vi "Main.vi"() -> ()   [LabVIEW 2022 SP3]
doc: "This template is for the Queued Message Handler design pattern.\n\nThe Event Handling Loop generates messages based on user interface actions.\n\nThe Message Handling Loop processes messages generated by the Event Handling Loop, or by other messages. The messages are string values, so new messages can be added easily to the Message Cases case structure in the Message Handling Loop. Each message cluster can also provide an optional value for Message Data, which is a variant that can be converted to whatever message-specific data is required."
uses:
  controls/UI Data.ctl
  controls/UI State.ctl
  controls/Config.ctl
  support/Message Queue/Enqueue Message (Single).vi
  support/Message Queue/Enqueue Message (Array).vi
  <vilib>/Utility/error.llb/Error Cluster From Error Code.vi
  <vilib>/ErrorRing/Error Ring.xnode
  support/Message Queue/Message Queue.lvlib
  support/User Event - Stop/User Event - Stop.lvlib
  Logging/Logging.lvlib
panel:
  out "PWM Value":dbl
  out "Temperature":dbl
  out "Stop":bool=TRUE
  out "Run":bool=TRUE
  out "PWM":dbl(knob) scale=0.0..255.0
  out "Hibák":errorcluster
  out "Waveform Chart":waveform(dbl)[](graph)
  out "Output":cluster{cluster{"Xi":dbl, "Yi":dbl}[]}[](graph)
  out "Error":cluster{cluster{"Xi":dbl, "Yi":dbl}[]}[](graph)
  out "Temperature":cluster{cluster{"Xi":dbl, "Yi":dbl}[]}[](graph)
  in  "Settings":bool
  out "Display":string
  in  "Stop":bool
  in  "Start":bool
  in  "Exit":bool
  # "°C"
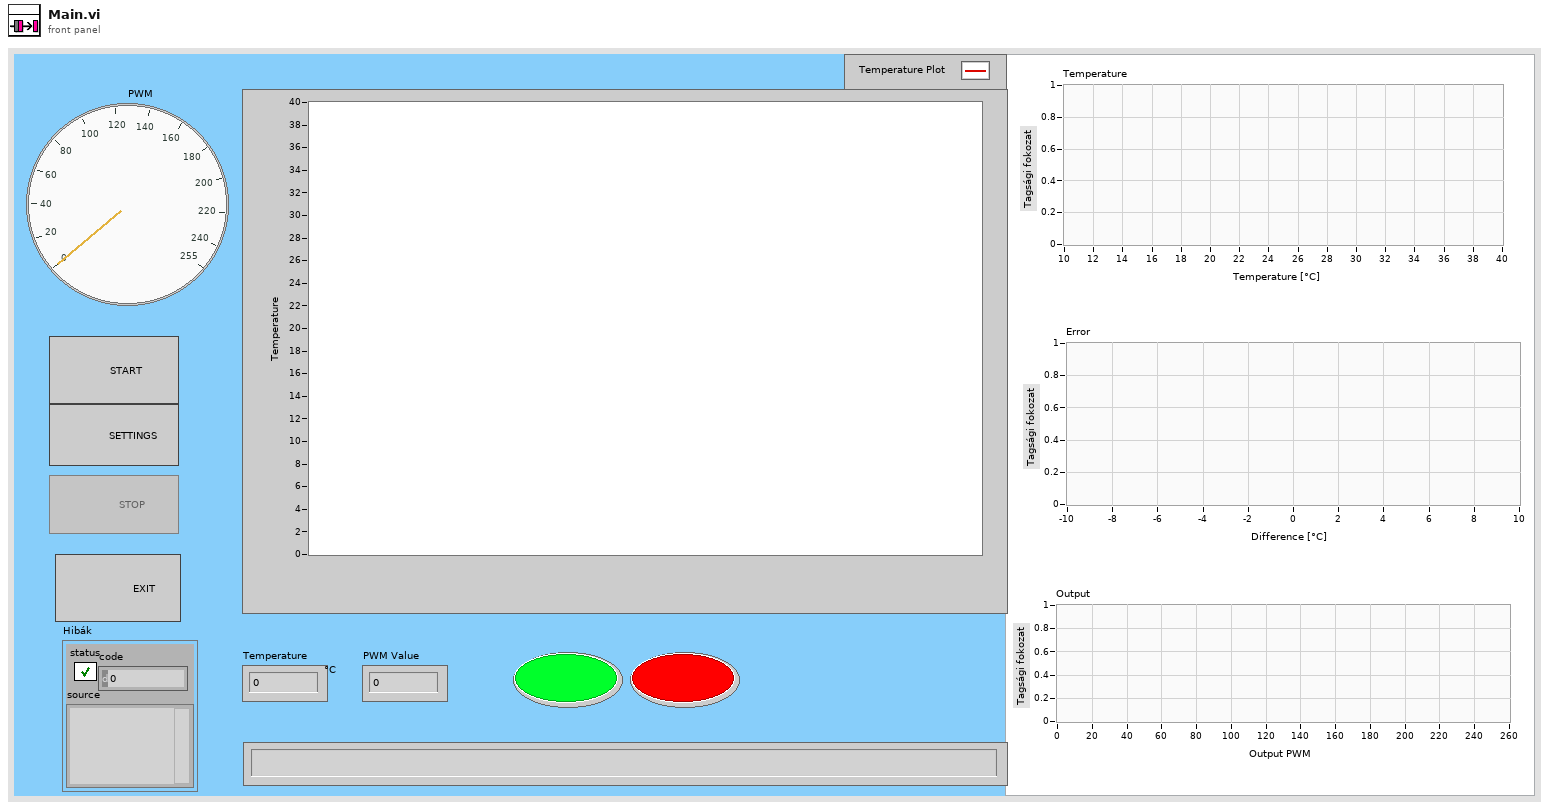
[diagram p1: front panel]
types:
  T1 = typedef "Config.ctl" = cluster{"Hardware":cluster{"VISA resource name":refnum<visa-resource-name>}, "Logging":cluster{"tdms file out":refnum<k34>, "base path":path}, "Set Temp":cluster{"Numeric":dbl}}
  T2 = typedef "UI State.ctl" = enum16{"Idle", "Acquiring and logging", "Waiting for Exit", "Waiting for Stop"}
  T3 = typedef "UI Data.ctl" = cluster{"Boolean <Replace Me>":bool, "String":string, "Numeric <Replace Me>":dbl, "Start ref":refnum<vi>, "Stop ref":refnum<vi>, "Data Display Ref":refnum<vi>, "Exit Button Ref":refnum<vi>, "Settings ref":refnum<vi>}
  T4 = typedef "Message Queue.lvlib/All Message Queues.ctl" = cluster{"UI":refnum<queue>, "Acquisition":refnum<queue>, "Logging":refnum<queue>}
  T5 = cluster{"Hardware":cluster{"VISA resource name":refnum<visa-resource-name>}, "Logging":cluster{"tdms file out":refnum<k34>, "base path":path}, "Set Temp":cluster{"Numeric":dbl}}
  T6 = cluster{"tdms file out":refnum<k34>, "base path":path}
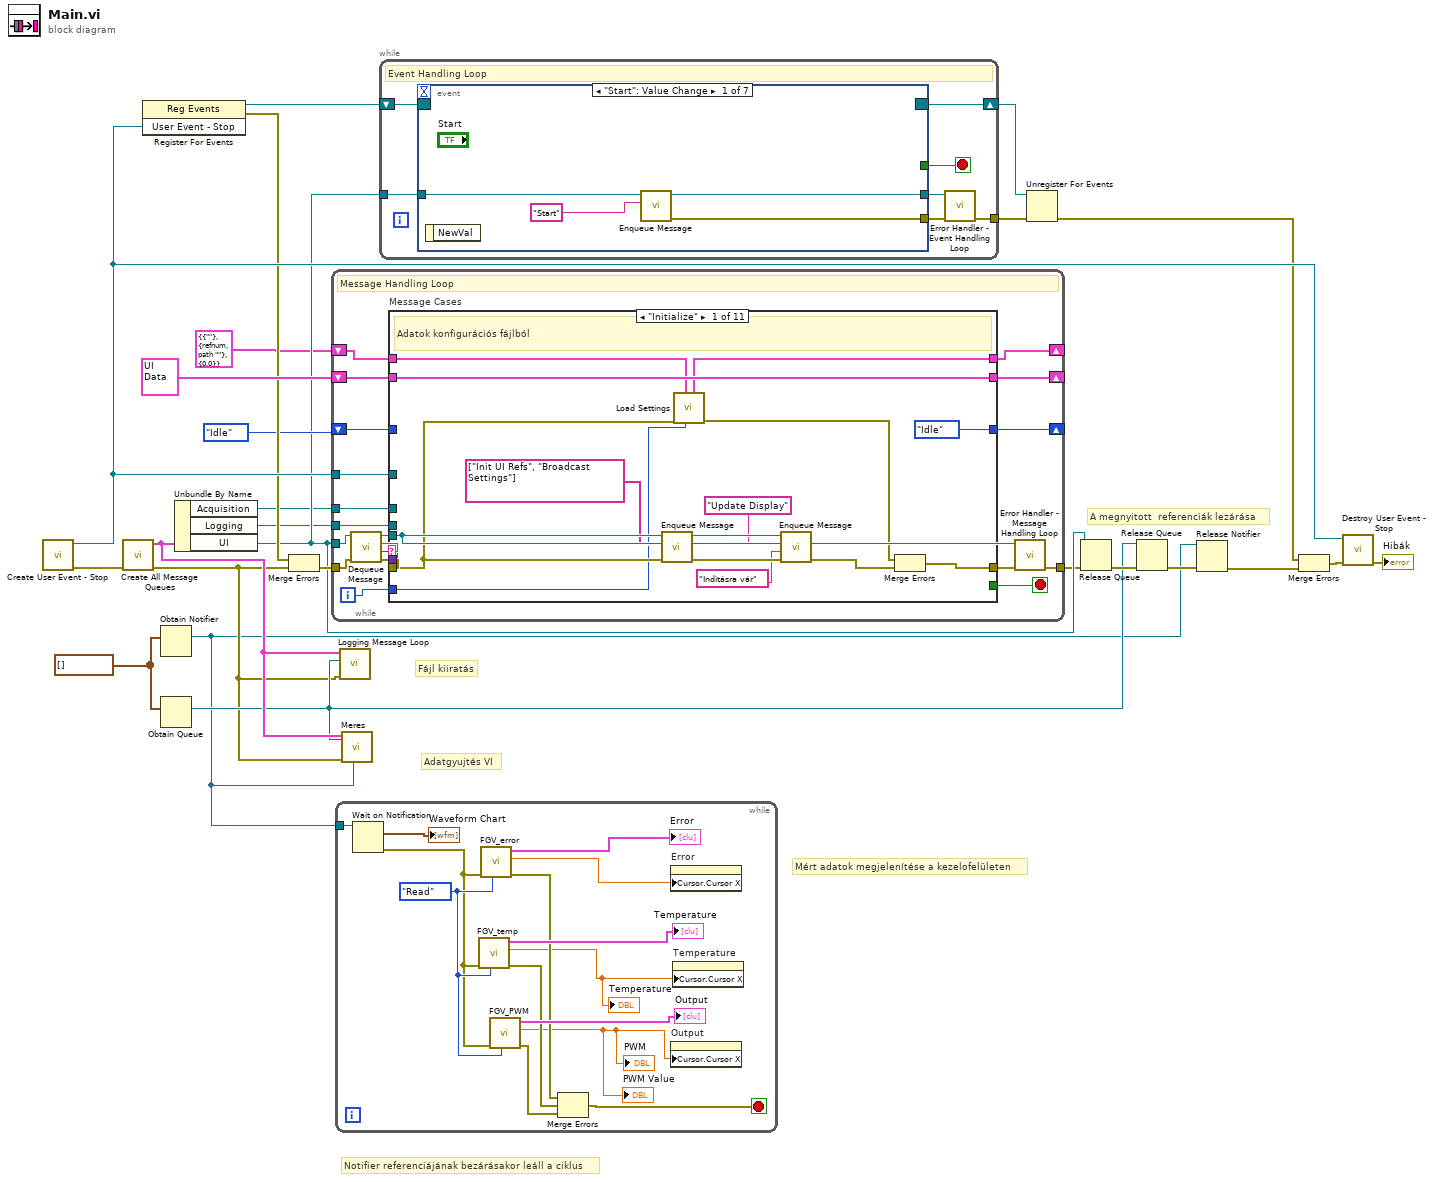
[diagram p0: block diagram]
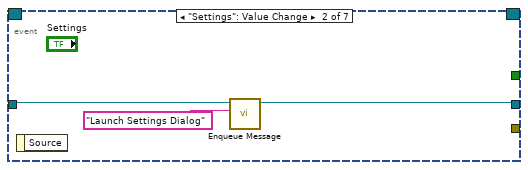
[diagram p2: hidden frame]
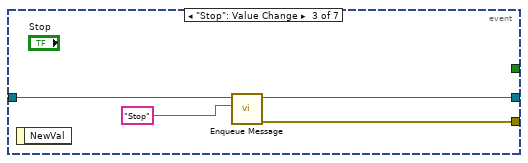
[diagram p3: hidden frame]
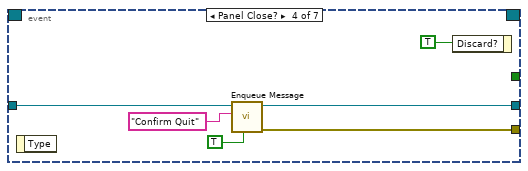
[diagram p4: hidden frame]
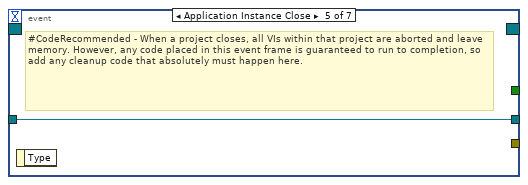
[diagram p5: hidden frame]
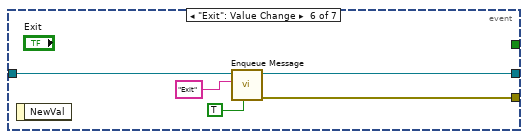
[diagram p6: hidden frame]
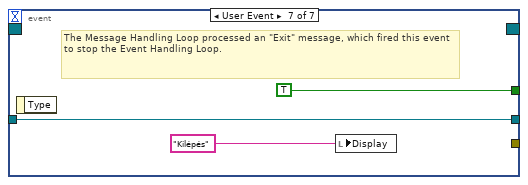
[diagram p7: hidden frame]
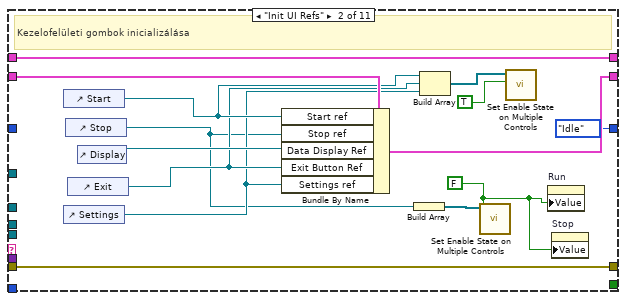
[diagram p8: hidden frame]
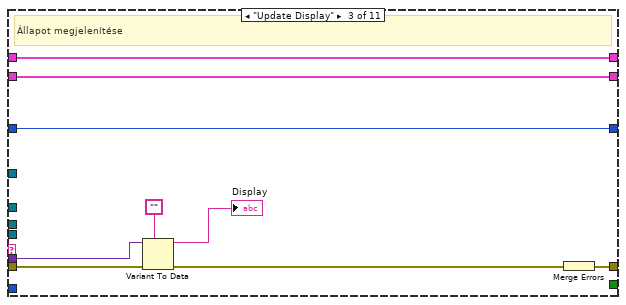
[diagram p9: hidden frame]
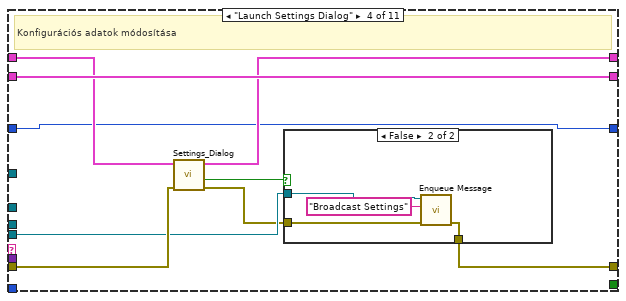
[diagram p10: hidden frame]
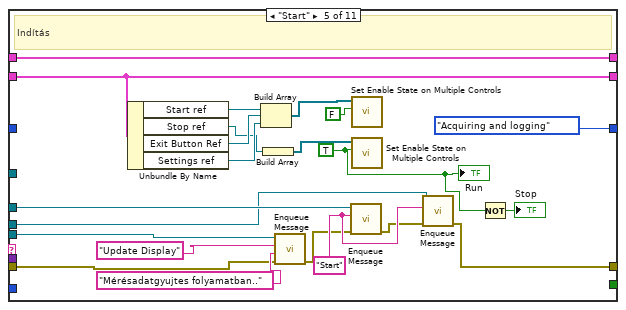
[diagram p12: hidden frame]
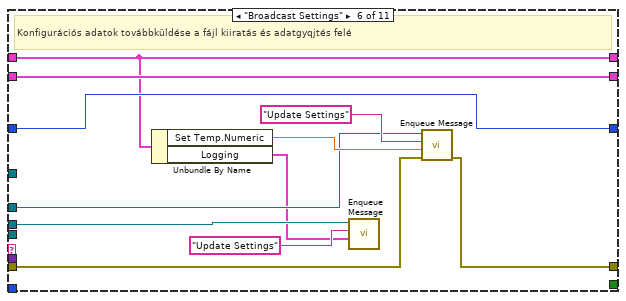
[diagram p13: hidden frame]
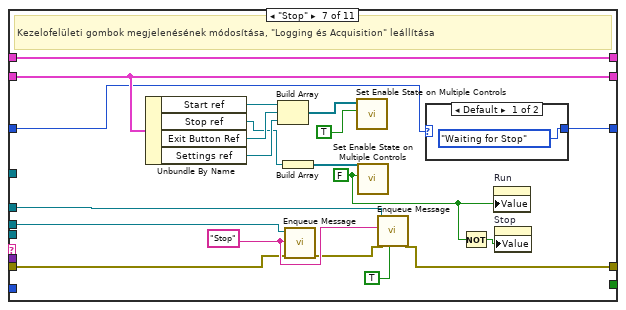
[diagram p14: hidden frame]
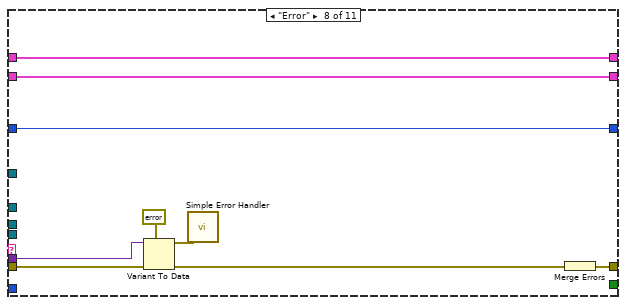
[diagram p16: hidden frame]
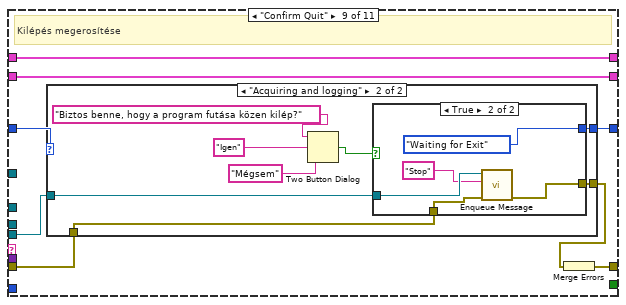
[diagram p17: hidden frame]
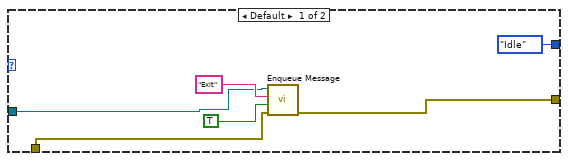
[diagram p18: hidden frame]
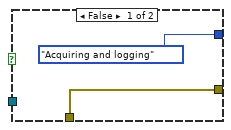
[diagram p19: hidden frame]
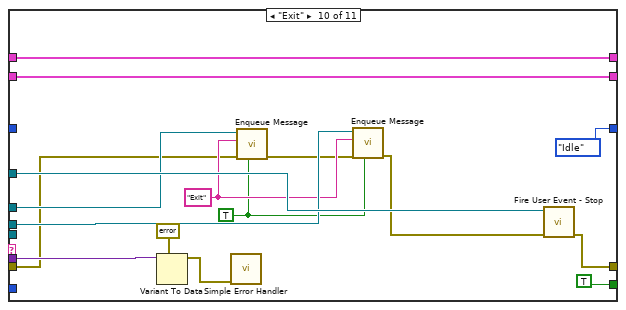
[diagram p20: hidden frame]
diagram:
  w9 = waveform(dbl)[] []
  # "Notifier referenciájának bezárásakor leáll a ciklus"
  # "Fájl kiiratás"
  # "Adatgyujtés VI"
  # "Mért adatok megjelenítése a kezelofelületen"
  # "A megnyitott  referenciák lezárása"
  n1 = call "Create User Event - Stop.vi"() -> ("error out"=w25:errorcluster, "User Event - Stop"=w19:refnum<user-event>)  [unwired: 10 in]
  n2 = call "Create All Message Queues.vi"("error in (no error)"=w25) -> ("error out"=w4:errorcluster, "Message Queues out"=w6:T4)  [unwired: 9 in]
  n3 = register-events(w19) -> (reference out=w20:refnum<event-registration>, error out=w17:errorcluster)  [unwired: 2 in]
  n4 = Obtain Notifier(notification data type=w9) -> (notifier out=w3:refnum<notifier>)  [unwired: 3 in, 2 out]
  n5 = Obtain Queue(element data type=w9) -> (queue out=w5:refnum<queue>)  [unwired: 4 in, 2 out]
  n6 = Unbundle By Name(w6) -> ("Acquisition"=w12:refnum<queue>, "Logging"=w11:refnum<queue>, "UI"=w15:refnum<queue>)
  n7 = Merge Errors(w17, w4) -> (w18:errorcluster)
  n8 = while {
    tunnel: w15 -> [w36]
    shift-right: [w43] -> _
    shift-left: T3 {"Boolean <Replace Me>"=FALSE, "String"="", "Numeric <Replace Me>"=0.0, "Start ref"=refnum, "Stop ref"=refnum, "Data Display Ref"=refnum, "Exit Button Ref"=refnum, "Settings ref"=refnum} ("Data Cluster") -> [w44]
    tunnel: w19 -> [w41]
    tunnel: w18 -> [w40]
    tunnel: [w34] -> w10
    shift-right: [w32] -> _
    shift-left: UI_State."Idle" -> [w31]
    shift-right: [w30] -> _
    shift-left: T1 {"Hardware"={"VISA resource name"=""}, "Logging"={"tdms file out"=refnum, "base path"=path ""}, "Set Temp"={"Numeric"=0.0}} -> [w29]
    tunnel: w12 -> [w28]
    tunnel: w11 -> [w27]
    i -> [w26]
    stop <- w42 stop-if-true
    # "Message Handling Loop"
    n9 = call "Dequeue Message.vi"("error in (no error)"=w40, "Message Queue"=w36) -> ("error out"=w39:errorcluster, "Message Data"=w37:variant, "Message"=w38:string, "dup Message Queue"=w35:refnum<queue>)  [unwired: 6 in]
    n10 = case "Message Cases" shown="\"Initialize\"" w38 {
      selector: w38 -> [_ _ _ _ _ _ _ _ _ _ w208]
      tunnel: w35 -> [w56 _ _ w86 w109 _ _ _ w164 _ _]
      tunnel: w39 -> [w48 w63 w80 w88 w106 w124 w136 w160 w162 w193 _]
      tunnel: [w47 w63 w81 w84 w99 w123 w134 w154 w167 w198 w209] -> w33
      tunnel: w44 -> [w59 w73 w82 w91 w118 w129 w149 w159 w168 w205 w210]
      tunnel: [w59 w64 w82 w91 w118 w129 w149 w159 w168 w205 w210] -> w43
      tunnel: [_ _ _ _ _ _ _ _ _ TRUE _] -> w42
      tunnel: w37 -> [_ _ w79 _ _ _ _ w158 _ w200 _]
      tunnel: w41 -> [_ _ _ _ _ _ _ _ _ w203 _]
      tunnel: [UI_State."Idle" UI_State."Idle" w74 w83 UI_State."Acquiring and logging" w128 w140 w153 w163 UI_State."Idle" w206] -> w32
      tunnel: w31 -> [_ _ w74 w83 _ w128 w141 w153 w165 _ w206]
      tunnel: [w49 w62 w75 w89 w105 w122 w139 w152 w166 w197 w207] -> w30
      tunnel: w29 -> [w50 w62 w75 w90 w105 w122 w139 w152 w166 w197 w207]
      tunnel: w28 -> [_ _ _ _ w104 w125 w138 _ _ w196 _]
      tunnel: w27 -> [_ _ _ _ w103 w121 w132 _ _ w195 _]
      tunnel: w26 -> [w45 _ _ _ _ _ _ _ _ _ _]
      frame "Initialize" {
        # "Adatok konfigurációs fájlból"
        n11 = call-poly "Enqueue Message.vi"("error in (no error)"=w48, "Message Array"=string[] ["Init UI Refs", "Broadcast Settings"], "Message Queue"=w56) -> ("error out"=w58:errorcluster, "dup Message Queue"=w55:refnum<queue>)  [unwired: 7 in]
        n12 = call "Load Settings.vi"("Elso?"=w45, "Config"=w50, "error constant"=w48) -> ("error constant 2"=w46:errorcluster, "Config 2"=w49:T5)  [unwired: 7 in]
        n13 = call-poly "Enqueue Message.vi"("error in (no error)"=w58, "Message Data"="Inditásra vár" ("Message"), "Message"="Update Display", "Message Queue"=w55) -> ("error out"=w57:errorcluster)  [unwired: 6 in, 1 out]
        n14 = Merge Errors(w46, w57) -> (w47:errorcluster)
      }
      frame "Init UI Refs" {
        w60 = FALSE ("Enable?")
        # "Kezelofelületi gombok inicializálása"
        n15 = control-ref of="Start"() -> (w71:refnum<vi>)
        n16 = control-ref of="Settings"() -> (w69:refnum<vi>)
        n17 = control-ref of="Stop"() -> (w68:refnum<vi>)
        n18 = control-ref of="Exit"() -> (w70:refnum<vi>)
        n19 = control-ref of="Display"() -> (w72:refnum<vi>)
        n20 = Bundle By Name(cluster=w73, "Start ref"=w71, "Stop ref"=w68, "Data Display Ref"=w72, "Exit Button Ref"=w70, "Settings ref"=w69) -> (w64:T3)
        n21 = Build Array(w68) -> (w67:refnum<vi>[])
        n22 = Build Array(w71, w70, w69) -> (w66:refnum<vi>[])
        n23 = call "Set Enable State on Multiple Controls.vi"("Enable?"=w60, "Controls"=w67) -> ()  [unwired: 10 in]
        n24 = call "Set Enable State on Multiple Controls.vi"("Enable?"=TRUE, "Controls"=w66) -> ()  [unwired: 10 in]
        n25 = property on="Run" class="Bool (strict)"("Value"=w60) -> ()  [unwired: 2 in, 2 out]
        n26 = property on="Stop" class="Bool (strict)"("Value"=w60) -> ()  [unwired: 2 in, 2 out]
      }
      frame "Update Display" {
        # "Állapot megjelenítése"
        n27 = Variant To Data(error in=w80, type="", Variant=w79) -> (data=→"Display":string, error out=w77:errorcluster)
        n28 = Merge Errors(w77) -> (w81:errorcluster)
      }
      frame "Launch Settings Dialog" {
        # "Konfigurációs adatok módosítása"
        n29 = call "Settings_Dialog.vi"("error IO 2"=w88, "Settings in"=w90) -> ("error IO"=w85:errorcluster, "Cancelled"=w87:bool, "Settings out"=w89:T1)  [unwired: 7 in]
        n30 = case shown="False" w87 {
          tunnel: w86 -> [_ w95]
          tunnel: w85 -> [w92 w94]
          tunnel: [w92 w93] -> w84
          frame True {
          }
          frame False {
            n31 = call-poly "Enqueue Message.vi"("error in (no error)"=w94, "Message"="Broadcast Settings", "Message Queue"=w95) -> ("error out"=w93:errorcluster)  [unwired: 7 in, 1 out]
          }
        }
      }
      frame "Start" {
        w102 = "Start" ("Message")
        w98 = TRUE ("Enable?")
        # "Indítás"
        n32 = Unbundle By Name(w118) -> ("Start ref"=w116:refnum<vi>, "Stop ref"=w111:refnum<vi>, "Exit Button Ref"=w115:refnum<vi>, "Settings ref"=w114:refnum<vi>)
        n33 = Build Array(w116, w115, w114) -> (w113:refnum<vi>[])
        n34 = Build Array(w111) -> (w112:refnum<vi>[])
        n35 = call-poly "Enqueue Message.vi"("error in (no error)"=w106, "Message Data"="Mérésadatgyujtes folyamatban.." ("Message"), "Message"="Update Display", "Message Queue"=w109) -> ("error out"=w101:errorcluster)  [unwired: 6 in, 1 out]
        n36 = call-poly "Enqueue Message.vi"("error in (no error)"=w101, "Message"=w102, "Message Queue"=w104) -> ("error out"=w100:errorcluster)  [unwired: 7 in, 1 out]
        n37 = call "Set Enable State on Multiple Controls.vi"("Enable?"=FALSE, "Controls"=w113) -> ()  [unwired: 10 in]
        n38 = call "Set Enable State on Multiple Controls.vi"("Enable?"=w98, "Controls"=w112) -> ()  [unwired: 10 in]
        n39 = call-poly "Enqueue Message.vi"("error in (no error)"=w100, "Message"=w102, "Message Queue"=w103) -> ("error out"=w99:errorcluster)  [unwired: 7 in, 1 out]
        n40 = Not(x=w98) -> (.not. x?=→"Stop":bool)
        "Run" <- w98
      }
      frame "Broadcast Settings" {
        # "Konfigurációs adatok továbbküldése a fájl kiiratás és adatgyqjtés felé"
        n41 = Unbundle By Name(w122) -> ("Set Temp.Numeric"=w127:dbl, "Logging"=w119:T6)
        n42 = call-poly "Enqueue Message.vi"("Message Data"=w119, "Message"="Update Settings", "Message Queue"=w121) -> ()  [unwired: 7 in, 2 out]
        n43 = call-poly "Enqueue Message.vi"("error in (no error)"=w124, "Message Data"=w127, "Message"="Update Settings", "Message Queue"=w125) -> ("error out"=w123:errorcluster)  [unwired: 6 in, 1 out]
      }
      frame "Stop" {
        w137 = "Stop" ("Message")
        w130 = FALSE ("Enable?")
        # "Kezelofelületi gombok megjelenésének módosítása, \"Logging és Acquisition\" leállítása"
        n44 = Unbundle By Name(w149) -> ("Start ref"=w148:refnum<vi>, "Stop ref"=w144:refnum<vi>, "Exit Button Ref"=w147:refnum<vi>, "Settings ref"=w146:refnum<vi>)
        n45 = Build Array(w148, w147, w146) -> (w145:refnum<vi>[])
        n46 = Build Array(w144) -> (w143:refnum<vi>[])
        n47 = call-poly "Enqueue Message.vi"("error in (no error)"=w136, "Message"=w137, "Message Queue"=w132) -> ("error out"=w135:errorcluster)  [unwired: 7 in, 1 out]
        n48 = call "Set Enable State on Multiple Controls.vi"("Enable?"=TRUE, "Controls"=w145) -> ()  [unwired: 10 in]
        n49 = call "Set Enable State on Multiple Controls.vi"("Enable?"=w130, "Controls"=w143) -> ()  [unwired: 10 in]
        n50 = call-poly "Enqueue Message.vi"("Priority Message? (F)"=TRUE, "error in (no error)"=w135, "Message"=w137, "Message Queue"=w138) -> ("error out"=w134:errorcluster)  [unwired: 6 in, 1 out]
        n51 = case shown="Default" w141 {
          selector: w141 -> [_ w151]
          tunnel: [UI_State."Waiting for Stop" w151] -> w140
          frame Default {
          }
          frame "Waiting for Exit" {
          }
        }
        n52 = Not(x=w130) -> (.not. x?=w131:bool)
        n53 = property on="Run" class="Bool (strict)"("Value"=w130) -> ()  [unwired: 2 in, 2 out]
        n54 = property on="Stop" class="Bool (strict)"("Value"=w131) -> ()  [unwired: 2 in, 2 out]
      }
      frame "Error" {
        n55 = Variant To Data(error in=w160, type=errorcluster {"status"=FALSE, "code"=0, "source"=""} ("error constant"), Variant=w158) -> (data=w156:errorcluster, error out=w155:errorcluster)
        n56 = call <vilib>:"Simple Error Handler.vi"("error in (no error)"=w156) -> ()  [unwired: 4 in, 5 out]
        n57 = Merge Errors(w155) -> (w154:errorcluster)
      }
      frame "Confirm Quit" {
        # "Kilépés megerosítése"
        n58 = case shown="\"Acquiring and logging\"" w165 {
          tunnel: w164 -> [w172 w178]
          tunnel: [UI_State."Idle" w177] -> w163
          tunnel: w162 -> [w170 w176]
          tunnel: [w169 w175] -> w161
          frame Default {
            n59 = call-poly "Enqueue Message.vi"("error in (no error)"=w170, "Message Data"=TRUE ("Priority Message? (F)"), "Message"="Exit", "Message Queue"=w172) -> ("error out"=w169:errorcluster)  [unwired: 6 in, 1 out]
          }
          frame "Acquiring and logging" {
            n60 = Two Button Dialog(message="Biztos benne, hogy a program futása közen kilép?", 1:"Mégsem" ("F button name (\"Cancel\")"), 2:"Igen" ("T button name (\"OK\")")) -> (T button?=w179:bool)
            n61 = case shown="True" w179 {
              tunnel: w178 -> [_ w189]
              tunnel: [UI_State."Acquiring and logging" UI_State."Waiting for Exit"] -> w177
              tunnel: [w183 w185] -> w175
              tunnel: w176 -> [w183 w186]
              frame False {
              }
              frame True {
                n62 = call-poly "Enqueue Message.vi"("error in (no error)"=w186, "Message"="Stop", "Message Queue"=w189) -> ("error out"=w185:errorcluster)  [unwired: 7 in, 1 out]
              }
            }
          }
        }
        n63 = Merge Errors(w161) -> (w167:errorcluster)
      }
      frame "Exit" {
        w190 = TRUE ("Priority Message? (F)")
        w194 = "Exit" ("Message")
        n64 = Variant To Data(type=errorcluster {"status"=FALSE, "code"=0, "source"=""} ("error constant"), Variant=w200) -> (data=w201:errorcluster)  [unwired: 1 in, 1 out]
        n65 = call <vilib>:"Simple Error Handler.vi"("error in (no error)"=w201) -> ()  [unwired: 4 in, 5 out]
        n66 = call-poly "Enqueue Message.vi"("Priority Message? (F)"=w190, "error in (no error)"=w193, "Message"=w194, "Message Queue"=w196) -> ("error out"=w192:errorcluster)  [unwired: 6 in, 1 out]
        n67 = call-poly "Enqueue Message.vi"("Priority Message? (F)"=w190, "error in (no error)"=w192, "Message"=w194, "Message Queue"=w195) -> ("error out"=w191:errorcluster)  [unwired: 6 in, 1 out]
        n68 = call "Fire User Event - Stop.vi"("error in (no error)"=w191, "User Event - Stop"=w203) -> ("error out"=w198:errorcluster)  [unwired: 9 in]
      }
      frame Default {
        n69 = xnode "Error Ring"("parameter 0"=w208) -> ("error out"=w209:errorcluster)
      }
    }
    n70 = call "Error Handler - Message Handling Loop.vi"("error in (no error)"=w33, "Message Queue"=w35) -> ("dup error in"=w34:errorcluster)  [unwired: 8 in, 1 out]
  }
  n71 = while {
    tunnel: w3 -> [w231]
    stop <- w220 stop-if-true
    w225 = enum16{"Read", "Write"}."Read" ("R/W")
    n72 = Wait on Notification(notifier=w231) -> (notification=→"Waveform Chart":waveform(dbl)[], error out=w224:errorcluster)  [unwired: 3 in, 2 out]
    n73 = call "FGV_temp.vi"("R/W"=w225, "error"=w224) -> ("error  out"=w222:errorcluster, "Value out"=w219:dbl, "Temp out"=→"Temperature":cluster{cluster{"Xi":dbl, "Yi":dbl}[]}[])  [unwired: 7 in]
    "Temperature" <- w219
    n74 = call "FGV_error.vi"("R/W"=w225, "error"=w224) -> ("error  out"=w223:errorcluster, "Value out"=w228:dbl, "FuzzyError out"=→"Error":cluster{cluster{"Xi":dbl, "Yi":dbl}[]}[])  [unwired: 7 in]
    n75 = call "FGV_PWM.vi"("R/W"=w225, "error"=w224) -> ("error  out"=w221:errorcluster, "Value out"=w218:dbl, "PWM out"=→"Output":cluster{cluster{"Xi":dbl, "Yi":dbl}[]}[])  [unwired: 7 in]
    "PWM" <- w218
    "PWM Value" <- w218
    n76 = Merge Errors(w223, w222, w221) -> (w220:errorcluster)
    n77 = property on="Error" class="XYGraph (strict)"("Cursor.Cursor X"=w228) -> ()  [unwired: 2 in, 2 out]
    n78 = property on="Output" class="XYGraph (strict)"("Cursor.Cursor X"=w218) -> ()  [unwired: 2 in, 2 out]
    n79 = property on="Temperature" class="XYGraph (strict)"("Cursor.Cursor X"=w219) -> ()  [unwired: 2 in, 2 out]
  }
  n80 = call "Logging Message Loop.vi"("error in (no error)"=w4, "Data Queue"=w5, "Message Queues"=w6) -> ()  [unwired: 8 in, 1 out]
  n81 = call "Meres.vi"("notifier"=w3, "queue"=w5, "error in"=w4, "Message Queues"=w6) -> ()  [unwired: 7 in, 1 out]
  n82 = while {
    tunnel: w15 -> [w238]
    shift-right: [w236] -> w23
    shift-left: w20 -> [w237]
    tunnel: [w232] -> w21
    stop <- w234 stop-if-true
    # "Event Handling Loop"
    n83 = event shown="[0] \"Start\": Value Change" {
      selector: w237 -> [_ _ _ _ _ _ _]
      dyn-events: [_ _ _ _ _ _ _] -> w236
      timeout: _ -> [_ _ _ _ _ _ _]
      tunnel: [_ _ _ _ _ _ TRUE ("Discard?")] -> w234
      tunnel: w238 -> [w242 w245 w249 w254 w256 w261 w264]
      tunnel: [w239 _ w246 w253 _ w260 _] -> w235
      tunnel: [w241 w243 w248 w252 w256 w259 w264] -> w233
      event "Start": Value Change {
        n84 = event-data() -> ()  [unwired: 1 in, 1 out]
        n85 = call-poly "Enqueue Message.vi"("Message"="Start", "Message Queue"=w242) -> ("error out"=w239:errorcluster, "dup Message Queue"=w241:refnum<queue>)  [unwired: 8 in]
      }
      event "Settings": Value Change {
        n86 = event-data() -> ()  [unwired: 1 in, 1 out]
        n87 = call-poly "Enqueue Message.vi"("Message"="Launch Settings Dialog", "Message Queue"=w245) -> ("dup Message Queue"=w243:refnum<queue>)  [unwired: 8 in, 1 out]
      }
      event "Stop": Value Change {
        n88 = event-data() -> ()  [unwired: 1 in, 1 out]
        n89 = call-poly "Enqueue Message.vi"("Message"="Stop", "Message Queue"=w249) -> ("error out"=w246:errorcluster, "dup Message Queue"=w248:refnum<queue>)  [unwired: 8 in]
      }
      event Panel Close? {
        n90 = event-data() -> ()  [unwired: 1 in, 1 out]
        n91 = call-poly "Enqueue Message.vi"("Priority Message? (F)"=TRUE, "Message"="Confirm Quit", "Message Queue"=w254) -> ("error out"=w253:errorcluster, "dup Message Queue"=w252:refnum<queue>)  [unwired: 7 in]
        n92 = event-data("Discard?"=TRUE) -> ()  [unwired: 1 in, 1 out]
      }
      event Application Instance Close {
        # "#CodeRecommended - When a project closes, all VIs within that project are aborted and leave memory. However, any code placed in this event frame is guaranteed to run to completion, so add any cleanup code that absolutely must happen here."
        n93 = event-data() -> ()  [unwired: 1 in, 1 out]
      }
      event "Exit": Value Change {
        n94 = event-data() -> ()  [unwired: 1 in, 1 out]
        n95 = call-poly "Enqueue Message.vi"("Priority Message? (F)"=TRUE, "Message"="Exit", "Message Queue"=w261) -> ("error out"=w260:errorcluster, "dup Message Queue"=w259:refnum<queue>)  [unwired: 7 in]
      }
      event User Event {
        # "The Message Handling Loop processed an \"Exit\" message, which fired this event to stop the Event Handling Loop."
        n96 = event-data() -> ()  [unwired: 1 in, 1 out]
        n97 = local write "Display"("Kilépés" ("VI Stopped")) -> ()
      }
    }
    n98 = call "Error Handler - Event Handling Loop.vi"("error in (no error)"=w235, "Message Queue"=w233) -> ("dup error in"=w232:errorcluster)  [unwired: 8 in, 1 out]
  }
  n99 = Unregister For Events(event registration refnum=w23, error in=w21) -> (error out=w14:errorcluster)
  n100 = Release Queue(queue=w15, error in (no error)=w10) -> (error out=w8:errorcluster)  [unwired: 1 in, 2 out]
  n101 = Release Queue(queue=w5, error in (no error)=w8) -> (error out=w7:errorcluster)  [unwired: 1 in, 2 out]
  n102 = Release Notifier(notifier=w3, error in (no error)=w7) -> (error out=w1:errorcluster)  [unwired: 1 in, 2 out]
  n103 = Merge Errors(w14, w1) -> (w24:errorcluster)
  n104 = call "Destroy User Event - Stop.vi"("error in (no error)"=w24, "User Event - Stop"=w19) -> ("error out"=→"Hibák":errorcluster)  [unwired: 9 in]
